vi "Execute.vi"(8 "error in (no error)":errorcluster, 11 "Generic Cmd in":refnum<class "Generic Cmd.lvclass">) -> (0 "error out":errorcluster, 3 "Generic Cmd out":refnum<class "Generic Cmd.lvclass">)   [LabVIEW 2020, in "Generic Actor.lvlib" / "Generic Cmd.lvclass"]
uses:
  Generic Cmd.lvclass
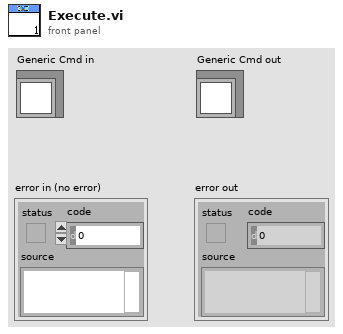
[diagram p1: front panel]
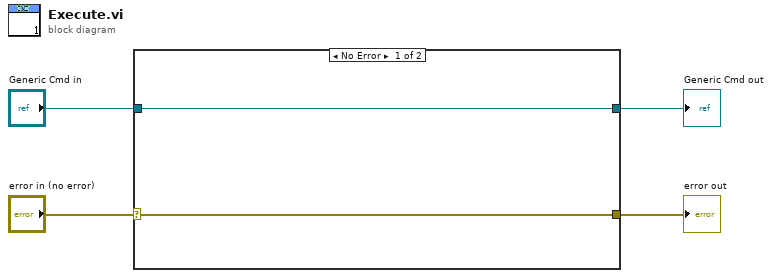
[diagram p0: block diagram]
diagram:
  n1 = case shown="No Error" "error in (no error)" {
    selector: "error in (no error)" -> [w5 w8]
    tunnel: [w5 w8] -> w3
    tunnel: [w6 w7] -> w1
    tunnel: "Generic Cmd in" -> [w6 w7]
    frame No Error {
    }
    frame Error {
    }
  }
  "error out" <- w3
  "Generic Cmd out" <- w1
